vi "demo_Debugging Enhancements in 2026.vi"(11 "Stop Demo":refnum<user-event>) -> ()   [LabVIEW 2020]
panel:
  # "LabVIEW 2026 Q1 - Debugging Enhancements\n\n- Set the Allow Debugging setting on all VIs under a target without modifying the VIs\n- Set and preserve Probes without modifying the source VI\n- Set and preserve Breakpoints without modifying the source VI"
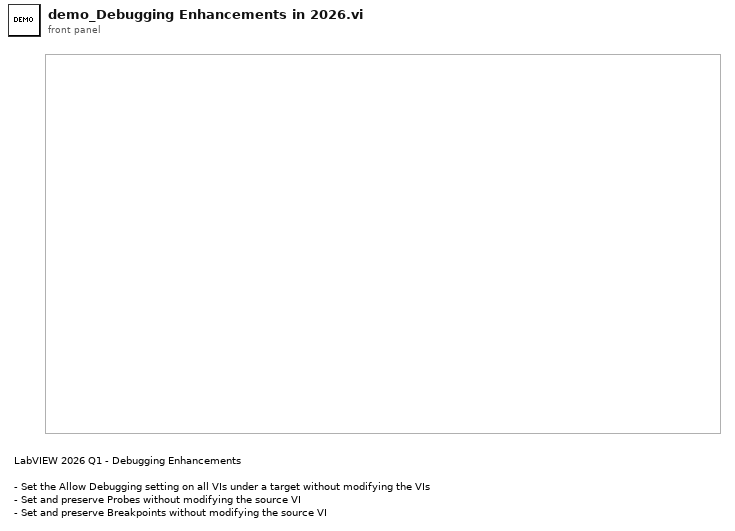
[diagram p1: front panel]
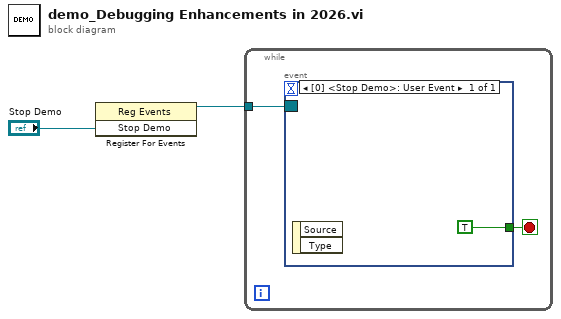
[diagram p0: block diagram]
diagram:
  n1 = register-events("Stop Demo") -> (reference out=w1:refnum<event-registration>)  [unwired: 2 in, 1 out]
  n2 = while {
    tunnel: w1 -> [w4]
    stop <- w3 stop-if-true
    n3 = event shown="[0] <Stop Demo>: User Event" {
      selector: w4 -> [_]
      dyn-events: _ -> [_]
      timeout: _ -> [_]
      tunnel: [TRUE] -> w3
      event User Event {
        n4 = event-data() -> ()  [unwired: 1 in, 2 out]
      }
    }
  }
